vi "Daq_Task_Factory.vi"(6 "Channel Names":string[](array[string]), 8 "error in":errorcluster, 9 "minimum value":dbl=-0.01 format="%^.2e", 10 "maximum value":dbl=0.01 format="%^.2e", 11 "DAQmx Physical Channels":tag[](array[tag])) -> (0 "error out":errorcluster, 3 "DAQmx Task Name":refnum<k21>)   [LabVIEW 2025]
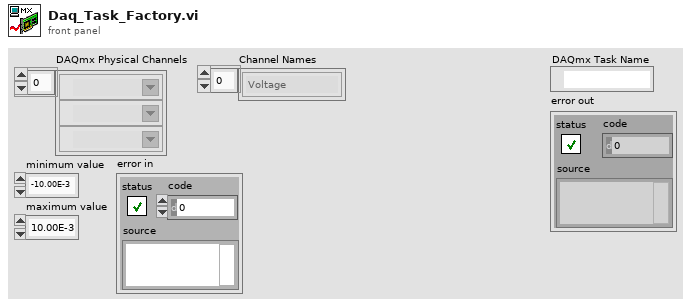
[diagram p1: front panel]
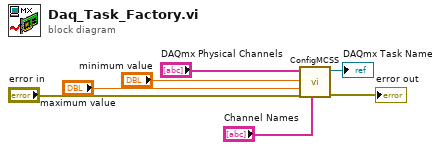
[diagram p0: block diagram]
diagram:
  n1 = call <vilib>:"ConfigMCSS.vi"("Channel Names"="Channel Names", "error in"="error in", "maximum value"="maximum value", "minimum value"="minimum value", "DAQmx Physical Channels"="DAQmx Physical Channels") -> ("error out"=→"error out":errorcluster, "DAQmx Task Name"=→"DAQmx Task Name":refnum<k21>)  [unwired: 5 in]
